vi "RCservo.vi"(8 "error in (no error)":errorcluster, 9 "Value":i32=1500, 10 "ID":i32, 11 "VISA resource name":refnum<visa-resource-name>) -> (0 "error out":errorcluster, 3 "VISA resource name out":refnum<visa-resource-name>)   [LabVIEW 2018]
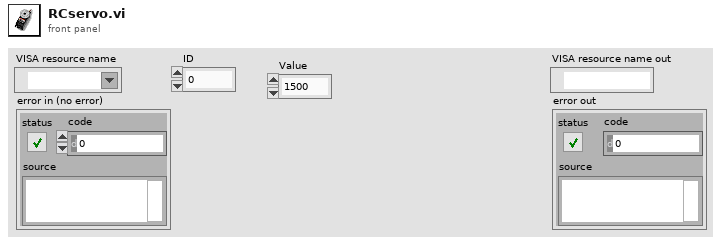
[diagram p1: front panel]
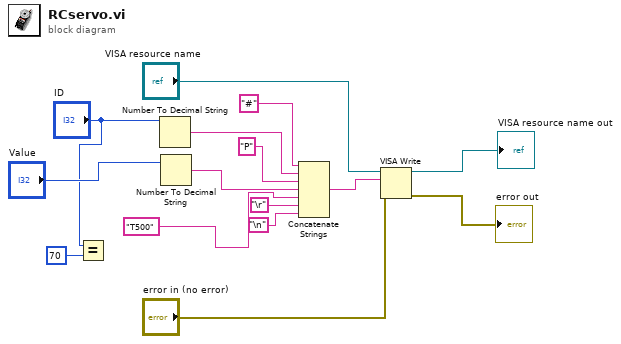
[diagram p0: block diagram]
diagram:
  n1 = Equal?(x="ID", y=70) -> ()  [unwired: 1 out]
  n2 = Number To Decimal String(number="ID") -> (decimal integer string=w6:string)  [unwired: 1 in]
  n3 = Number To Decimal String(number="Value") -> (decimal integer string=w4:string)  [unwired: 1 in]
  n4 = Concatenate Strings("#" ("string"), w6, "P" ("string"), w4, "T500" ("string"), "\r", "\n") -> (w15:string)
  n5 = VISA Write(VISA resource name="VISA resource name", write buffer=w15, error in (no error)="error in (no error)") -> (VISA resource name out=→"VISA resource name out":refnum<visa-resource-name>, error out=→"error out":errorcluster)  [unwired: 1 out]
